vi "ExtractTaskChannels.vi"(8 "error in (no error)":errorcluster, 9 "Board Data":u32[](array[numeric]), 10 "Preamp Data":u32[](array[numeric]), 11 "IntanElectrophysiology in":refnum<class "IntanElectrophysiology.lvclass">) -> (0 "error out":errorcluster, 2 "Extracted Data":i32[][](array[numeric]), 3 "IntanElectrophysiology out":refnum<class "IntanElectrophysiology.lvclass">)   [LabVIEW 2014, in "IntanElectrophysiology.lvclass"]
uses:
  IntanElectrophysiology.lvclass
  IntanElectrophysiology.lvclass/IntanElectrophysiology.ctl
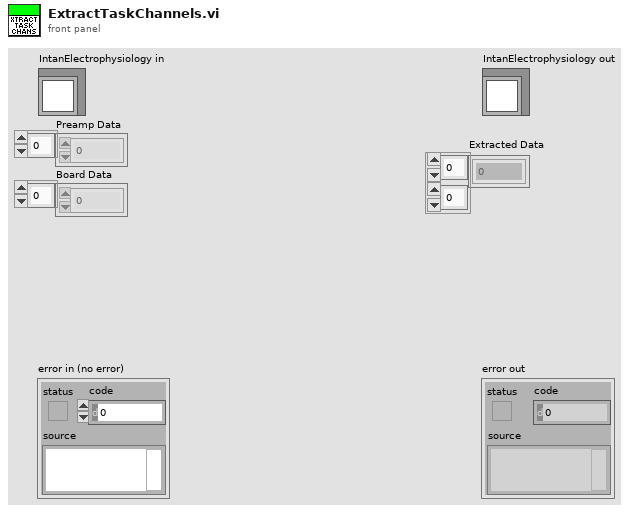
[diagram p1: front panel]
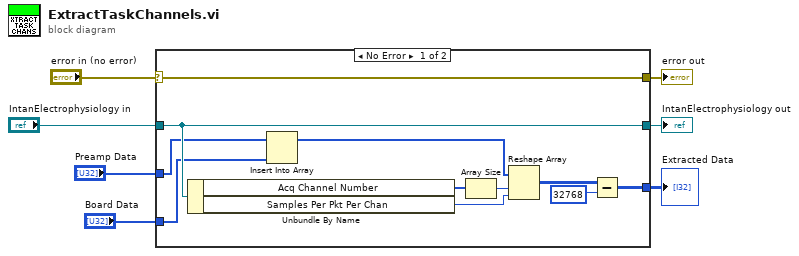
[diagram p0: block diagram]
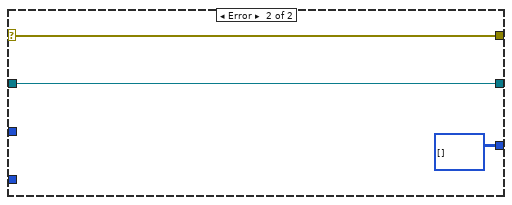
[diagram p2: hidden frame]
diagram:
  n1 = case shown="No Error" "error in (no error)" {
    selector: "error in (no error)" -> [w18 w21]
    tunnel: [w18 w21] -> w6
    tunnel: [w17 w20] -> w4
    tunnel: "IntanElectrophysiology in" -> [w17 w20]
    tunnel: "Preamp Data" -> [w9 _]
    tunnel: [w15 i32[][] []] -> w2
    tunnel: "Board Data" -> [w8 _]
    frame No Error {
      n2 = Unbundle By Name(w17) -> ("Acq Channel Number"=w13:i32[], "Samples Per Pkt Per Chan"=w11:i32)
      n3 = Insert Into Array(array=w9, new element=w8) -> (w14:u32[])  [unwired: 1 in]
      n4 = Array Size(array=w13) -> (size(s)=w12:i32)
      n5 = Reshape Array(w14, w12, w11) -> (w10:u32[][])
      n6 = Subtract(x=w10, y=32768) -> (x-y=w15:u32[][])
    }
    frame Error {
    }
  }
  "error out" <- w6
  "IntanElectrophysiology out" <- w4
  "Extracted Data" <- w2
